vi "CRYSend Curve Changing Event.vi"(11 "Type":enum16{"Curves", "Values", "Results", "WFM"}[](array[ring])) -> ()   [LabVIEW 2013]
uses:
  CRYStepSetup Global.vi
panel:
  # "Send Curve Library Change Event to current edit step"
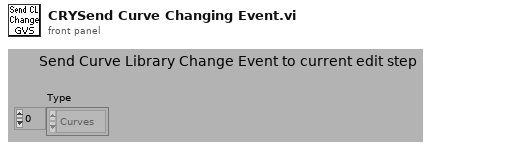
[diagram p1: front panel]
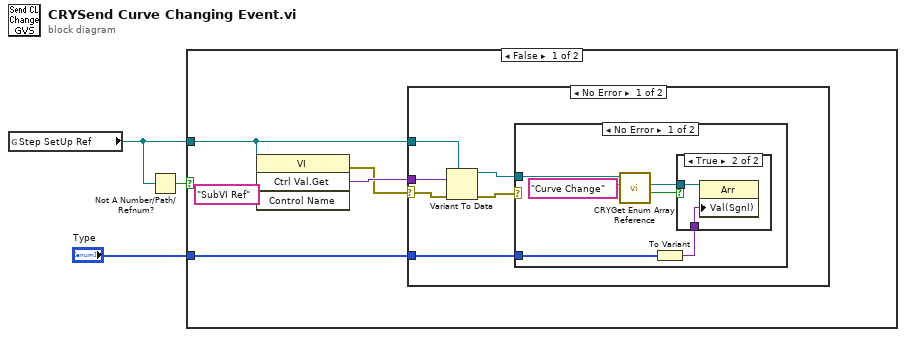
[diagram p0: block diagram]
diagram:
  n1 = global read "CRYStepSetup Global.vi" "Step SetUp Ref"() -> (w2:refnum<vi>)
  n2 = Not A Number/Path/Refnum?(number/path/refnum=w2) -> (NaN/Path/Refnum?=w1:bool)
  n3 = case shown="False" w1 {
    tunnel: "Type" -> [w8 _]
    tunnel: w2 -> [w5 _]
    frame False {
      n4 = invoke class="VI" method="Ctrl Val.Get"(reference=w5, "Control Name"="SubVI Ref") -> (error out=w4:errorcluster, "Get Control Value Variant"=w6:variant)  [unwired: 2 in, 2 out]
      n5 = case shown="No Error" w4 {
        selector: w4 -> [w10 _]
        tunnel: w6 -> [w14 _]
        tunnel: w5 -> [w13 _]
        tunnel: w8 -> [w11 _]
        frame No Error {
          n6 = Variant To Data(error in=w10, type=w13, Variant=w14) -> (data=w12:refnum<vi>, error out=w9:errorcluster)
          n7 = case shown="No Error" w9 {
            tunnel: w12 -> [w20 _]
            tunnel: w11 -> [w17 _]
            frame No Error {
              n8 = call "CRYGet Enum Array Reference.vi"("Label Name"="Curve Change", "VI Refnum"=w20) -> ("Boolean"=w15:bool, "Enum Array Ref Out"=w18:refnum<vi>)  [unwired: 8 out]
              n9 = To Variant(anything=w17) -> (Variant=w16:variant)
              n10 = case shown="True" w15 {
                tunnel: w18 -> [_ w22]
                tunnel: w16 -> [_ w21]
                frame False {
                }
                frame True {
                  n11 = property class="Arr"(reference=w22, "Val(Sgnl)"=w21) -> ()  [unwired: 1 in, 2 out]
                }
              }
            }
            frame Error {
            }
          }
        }
        frame Error {
        }
      }
    }
    frame True {
    }
  }
